vi "UpdateChart.vi"(8 "error in (no error)":errorcluster, 10 "Update Chart?":bool, 11 "DisplayWaveforms":refnum<class "DisplayWaveforms.lvclass">) -> (0 "error out":errorcluster, 3 "DisplayWaveforms out":refnum<class "DisplayWaveforms.lvclass">)   [LabVIEW 2018, in "DisplayWaveform.lvlib" / "DisplayWaveforms.lvclass"]
doc: "Update charts"
uses:
  DisplayWaveforms.lvclass
panel:
  # "For instructions on how to use the JKI State Machine Objects, examples and video tutorials, visit:\nhttp://jki.net/state-machine-objects/\n\nJKI State Machine Objects™\nhttp://jki.net/state-machine-objects/\nCopyright (C) 2005-2015, JKI <info@jki.net>\nALL RIGHTS RESERVED"
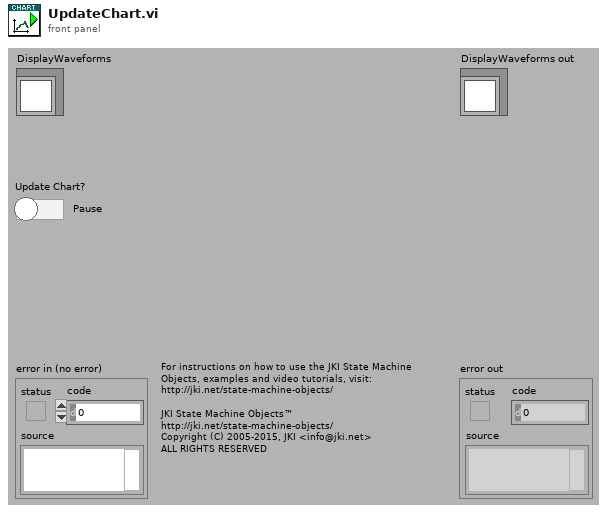
[diagram p1: front panel]
types:
  T1 = typedef "DisplayWaveform.lvlib/DisplayWaveforms.lvclass/ProtectedEvents--Cluster.ctl" = cluster{"Clear Chart":refnum<user-event>, "Pause Chart":refnum<user-event>, "Update Chart":refnum<user-event>, "Export Chart":refnum<user-event>, "Set ChartParams":refnum<user-event>}
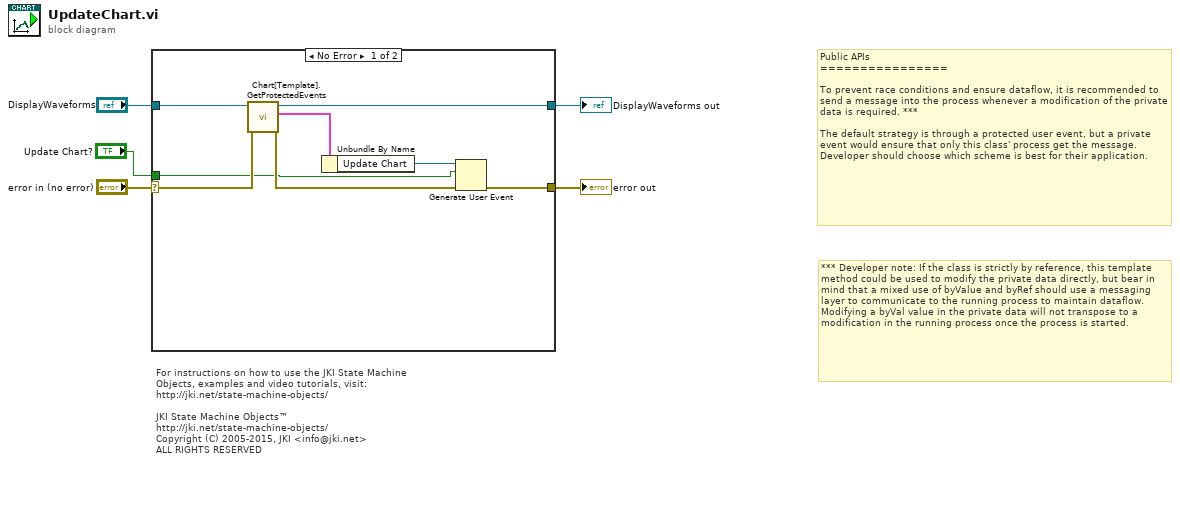
[diagram p0: block diagram]
diagram:
  # "*** Developer note: If the class is strictly by reference, this template method could be used to modify the private data directly, but bear in mind that a mixed use of byValue and byRef should use a messaging layer to communicate to the running process to maintain dataflow. Modifying a byVal value in the private data will not transpose to a modification in the running process once the process is started."
  # "Public APIs\n================\n\nTo prevent race conditions and ensure dataflow, it is recommended to send a message into the process whenever a modification of the private data is required. ***\n\nThe default strategy is through a protected user event, but a private event would ensure that only this class' process get the message. Developer should choose which scheme is best for their application."
  # "For instructions on how to use the JKI State Machine Objects, examples and video tutorials, visit:\nhttp://jki.net/state-machine-objects/\n\nJKI State Machine Objects™\nhttp://jki.net/state-machine-objects/\nCopyright (C) 2005-2015, JKI <info@jki.net>\nALL RIGHTS RESERVED"
  n1 = case shown="No Error" "error in (no error)" {
    selector: "error in (no error)" -> [w13 w14]
    tunnel: "DisplayWaveforms" -> [w10 w15]
    tunnel: [w12 w14] -> w4
    tunnel: [w11 w15] -> w3
    tunnel: "Update Chart?" -> [w6 _]
    frame No Error {
      n2 = call "Chart[Template].GetProtectedEvents.vi"("error in (no error)"=w13, "DisplayWaveforms"=w10) -> ("error out"=w7:errorcluster, "Protected Events"=w8:T1, "DisplayWaveforms out"=w11:refnum<class "DisplayWaveforms.lvclass">)  [unwired: 7 in]
      n3 = Unbundle By Name(w8) -> ("Update Chart"=w9:refnum<user-event>)
      n4 = Generate User Event(user event=w9, event data cluster=w6, error in=w7) -> (error out=w12:errorcluster)  [unwired: 1 in, 1 out]
    }
    frame Error {
    }
  }
  "error out" <- w4
  "DisplayWaveforms out" <- w3
